vi "Load Pattern.vi"(8 "error in (no error)":errorcluster, 10 "PatternData":T1(array[cluster]), 11 "CS++PPG in":refnum<class "CS++PPG.lvclass">) -> (0 "error out":errorcluster, 3 "CS++PPG out":refnum<class "CS++PPG.lvclass">)   [LabVIEW 2015, in "CS++PPG.lvlib" / "CS++PPG.lvclass"]
doc: "This VI loads a pattern to the pulsed pattern generator. Afterwards the PPG device should be ready to start."
uses:
  CS++PPG.lvclass
  CSPP_Core/Classes/CS++ProcessVariables/ProcessVariable/PV.lvclass
  PV-Enum.ctl
  CS++PPG.lvclass/CS++PPG.ctl
  CSPP_Core/Classes/CS++ProcessVariables/ProcessVariable/PV.lvclass/PV.ctl
  CSPP_Core/Classes/CS++ProcessVariables/ProcessVariable/Write Data.vi
  CSPP_Core/Classes/CS++ProcessVariables/ProcessVariable/Write Timestamp.vi
  CSPP_Core/Classes/CS++ProcessVariables/ProcessVariable/Write Quality.vi
  CSPP_Core/Classes/CS++ProcessVariables/ProcessVariable/Write status.vi
  CSPP_Core/Classes/CS++ProcessVariables/PVConnection/PVConnection.lvclass
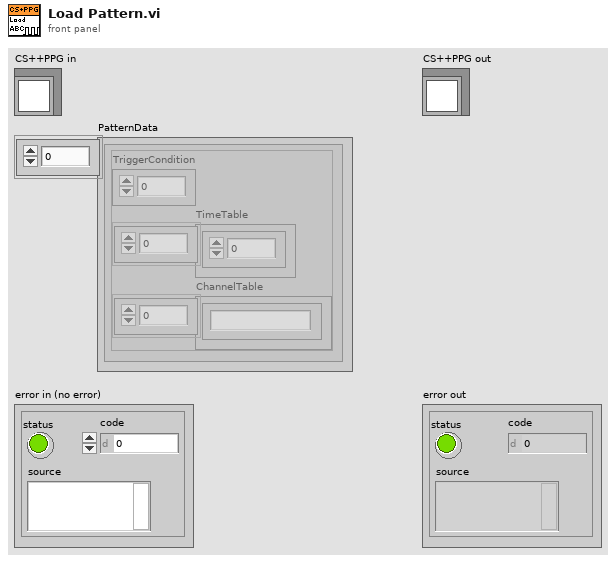
[diagram p1: front panel]
types:
  T1 = cluster{"TriggerCondition":i32, "TimeTable":dbl[], "ChannelTable":string[]}[]
  T2 = typedef "CS++PPG.lvlib/CS++PPG.lvclass/PV-Enum.ctl" = enum16{"Mode", "Trigger"}
  T3 = cluster{"TriggerCondition":i32, "TimeTable":dbl[], "ChannelTable":string[]}
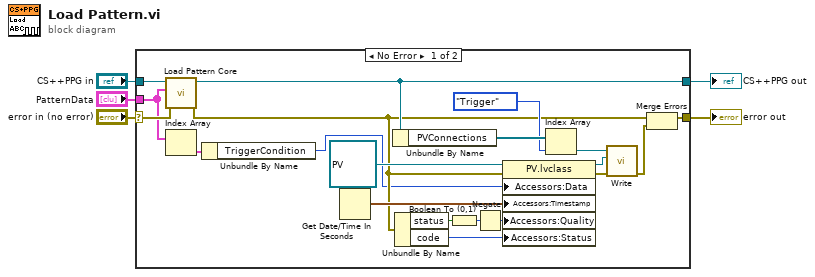
[diagram p0: block diagram]
diagram:
  n1 = case shown="No Error" "error in (no error)" {
    selector: "error in (no error)" -> [w24 w27]
    tunnel: [w10 w27] -> w4
    tunnel: [w11 w26] -> w2
    tunnel: "CS++PPG in" -> [w25 w26]
    tunnel: "PatternData" -> [w8 _]
    frame No Error {
      n2 = call-dynamic "Load Pattern Core.vi"("error in (no error)"=w24, "PatternData"=w8, "CS++PPG in"=w25) -> ("error out"=w9:errorcluster, "CS++PPG out"=w11:refnum<class "CS++PPG.lvclass">)  [unwired: 7 in]
      n3 = Index Array(array=w8) -> (element=w7:T3)  [unwired: 1 in]
      n4 = Unbundle By Name(w7) -> ("TriggerCondition"=w6:i32)
      n5 = Get Date/Time In Seconds() -> (seconds since 1Jan1904=w23:timestamp)
      n6 = Unbundle By Name(w11) -> ("PVConnections"=w15:refnum<class "PVConnection.lvclass">[])
      n7 = Unbundle By Name(w9) -> ("status"=w18:bool, "code"=w21:i32)
      n8 = Boolean To (0,1)(Boolean=w18) -> (0, 1=w20:i16)
      n9 = Negate(x=w20) -> (-x=w19:i16)
      n10 = property class="PV.lvclass"(reference=refnum<class "PV.lvclass"> refnum ("PV"), error in=w9, "Accessors:Data"=w6, "Accessors:Timestamp"=w23, "Accessors:Quality"=w19, "Accessors:Status"=w21) -> (reference out=w17:refnum<class "PV.lvclass">, error out=w16:errorcluster)
      n11 = Index Array(array=w15, index=PV-Enum."Trigger" ("PV-Enum")) -> (element=w14:refnum<class "PVConnection.lvclass">)
      n12 = call "Write.vi"("error in (no error)"=w16, "PV"=w17, "PVConnection in"=w14) -> ("error out"=w13:errorcluster)  [unwired: 7 in, 1 out]
      n13 = Merge Errors(w9, w13) -> (w10:errorcluster)
    }
    frame Error {
    }
  }
  "error out" <- w4
  "CS++PPG out" <- w2
